vi "Find Message Text.vi"(7 "Event Selector Name":string, 8 "error in (no error)":errorcluster, 11 "EventStructure in":refnum<vi>) -> (0 "error out":errorcluster, 5 "Message Text":string)   [LabVIEW 2017, in "Open DQMH Request Message Diagram.lvlib"]
doc: "Returns the Message text pass from the EHL to the MHL for the event handle by the Event Selectore Name event case."
uses:
  Open DQMH Request Message Diagram.lvlib
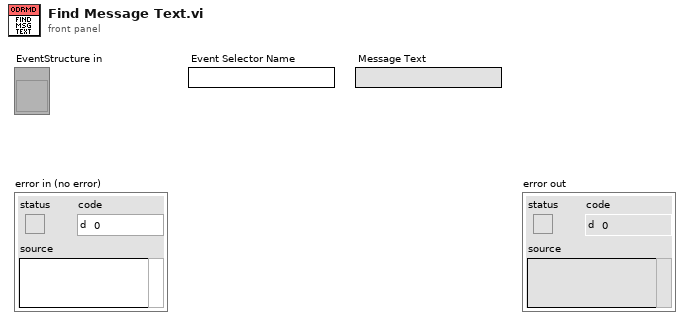
[diagram p1: front panel]
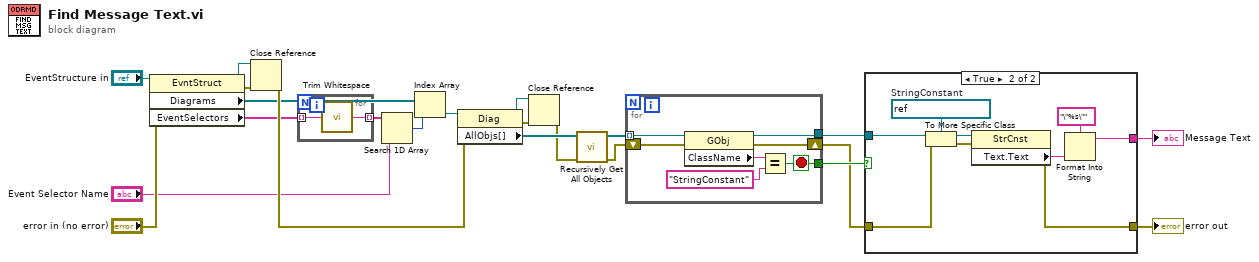
[diagram p0: block diagram]
diagram:
  n1 = property class="EvntStruct"(reference="EventStructure in", error in="error in (no error)") -> (reference out=w18:refnum<vi>, error out=w19:errorcluster, "Diagrams"=w16:refnum<vi>[], "EventSelectors"=w10:string[])
  n2 = Close Reference(reference=w18, error in (no error)=w19) -> (error out=w20:errorcluster)
  n3 = for {
    tunnel: w10 -> [w24] mode=indexing
    tunnel: [w23] -> w11 mode=indexing
    n4 = call <vilib>:"Trim Whitespace.vi"("string"=w24) -> ("trimmed string"=w23:string)  [unwired: 1 in]
  }
  n5 = Search 1D Array(1D array=w11, element="Event Selector Name") -> (index of element=w8:i32)  [unwired: 1 in]
  n6 = Index Array(array=w16, index=w8) -> (element=w9:refnum<vi>)
  n7 = property class="Diag"(reference=w9, error in=w20) -> (reference out=w5:refnum<vi>, error out=w21:errorcluster, "AllObjs[]"=w4:refnum<vi>[])
  n8 = Close Reference(reference=w5, error in (no error)=w21) -> (error out=w2:errorcluster)
  n9 = call "Recursively Get All Objects.vi"("error in (no error)"=w2, "AllObjs[] in"=w4) -> ("error out"=w1:errorcluster, "AllObjs[] out"=w3:refnum<vi>[])  [unwired: 8 in]
  n10 = for {
    tunnel: w3 -> [w26] mode=indexing
    tunnel: [w30] -> w12
    shift-right: [w28] -> w17
    shift-left: w1 -> [w29]
    tunnel: [w27] -> w22
    stop <- w27 stop-if-true
    n11 = property class="GObj"(reference=w26, error in=w29) -> (reference out=w30:refnum<vi>, error out=w28:errorcluster, "ClassName"=w25:string)
    n12 = Equal?(x=w25, y="StringConstant" ("Class Name")) -> (x = y?=w27:bool)
  }
  n13 = case shown="True" w22 {
    tunnel: w12 -> [_ w33]
    tunnel: [_ w37] -> w6
    tunnel: [w32 w36] -> w13
    tunnel: w17 -> [w32 w35]
    frame False {
    }
    frame True {
      w41 = refnum<vi> refnum  # StringConstant
      n14 = To More Specific Class(target class=w41, reference=w33, error in=w35) -> (specific class reference=w40:refnum<vi>, error out=w34:errorcluster)
      n15 = property class="StrCnst"(reference=w40, error in=w34) -> (error out=w36:errorcluster, "Text.Text"=w39:string)  [unwired: 1 out]
      n16 = Format Into String(format string="\"%s\"", w39) -> (resulting string=w37:string)  [unwired: 2 in, 1 out]
    }
  }
  "error out" <- w13
  "Message Text" <- w6
